vi "PF_FindExtrema.vi"(7 "Min Cut-off":sgl=0.25, 8 "Max Cut-on":sgl=0.75, 10 "Intensity Array":sgl[](array[numeric])) -> (1 "Extrema Array":T1(array[cluster]))   [LabVIEW 2019]
panel:
  in  "Extrema Cluster":T2={"type"=enum."maximum", "x"=0, "y"=0.0} {"y" format="%.2f"}
  # "Phase Fitter: Find Extrema"
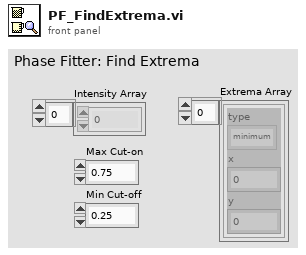
[diagram p1: front panel]
types:
  T1 = cluster{"type":enum16{"minimum", "maximum"}, "x":i32, "y":dbl}[]
  T2 = cluster{"type":enum16{"minimum", "maximum"}, "x":i32, "y":dbl}
  T3 = cluster{"Extremum":enum16{"minimum", "maximum"}, i32, sgl}
  T4 = cluster{"Extremum":enum16{"minimum", "maximum"}, "x":i32, "y":dbl}[]
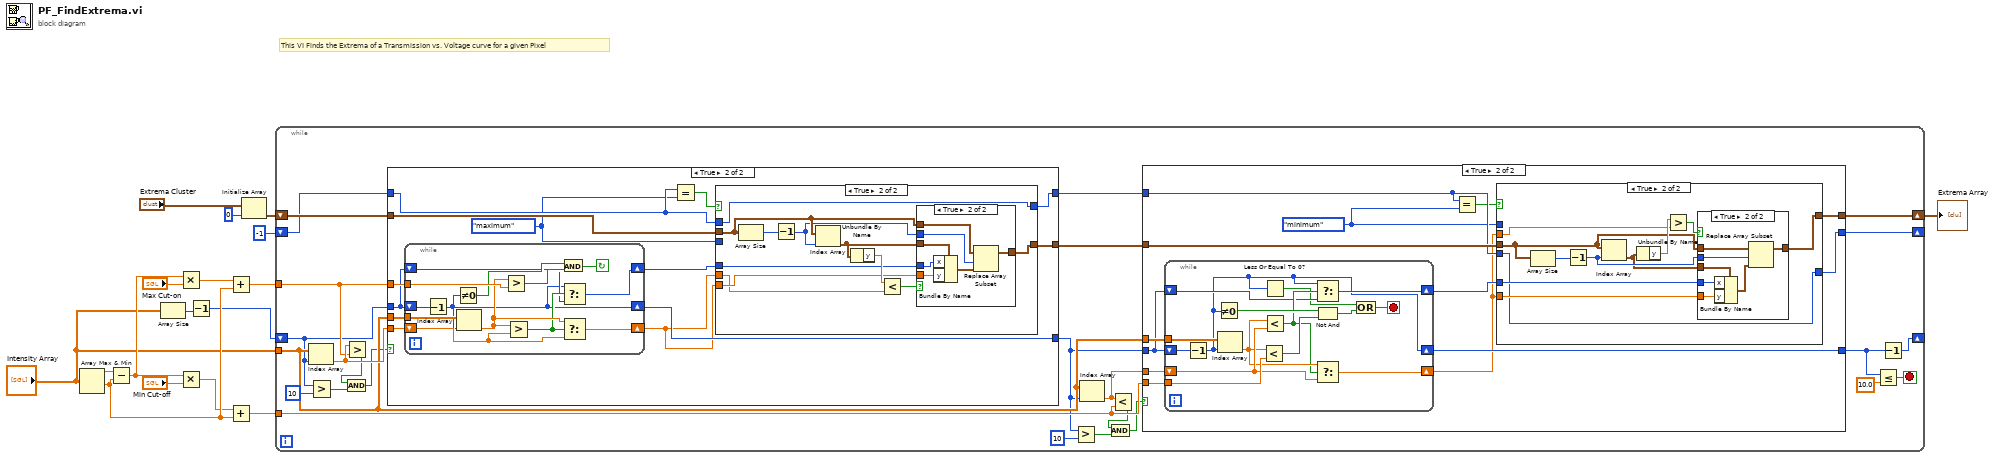
[diagram p0: block diagram]
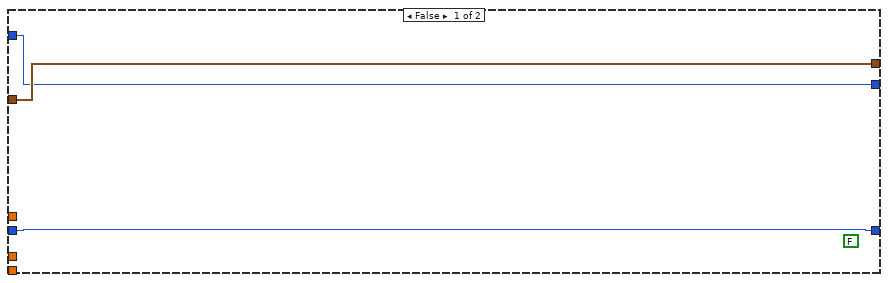
[diagram p2: hidden frame]
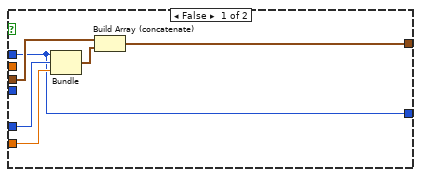
[diagram p3: hidden frame]
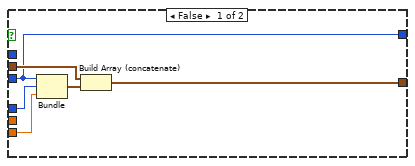
[diagram p6: hidden frame]
diagram:
  # "This VI Finds the Extrema of a Transmission vs. Voltage curve for a given Pixel"
  n1 = Array Max & Min(array="Intensity Array") -> (max value=w11:sgl, min value=w15:sgl)  [unwired: 2 out]
  n2 = Subtract(x=w11, y=w15) -> (x-y=w14:sgl)
  n3 = Array Size(array="Intensity Array") -> (size(s)=w3:i32)
  n4 = Multiply(x=w14, y="Max Cut-on") -> (x*y=w12:sgl)
  n5 = Multiply(x=w14, y="Min Cut-off") -> (x*y=w13:sgl)
  n6 = Decrement(x=w3) -> (x-1=w2:i32)
  n7 = Add(x=w12, y=w15) -> (x+y=w10:sgl)
  n8 = Add(x=w13, y=w15) -> (x+y=w9:sgl)
  n9 = Initialize Array("Extrema Cluster", 0 ("Dimension Size")) -> (w16:T1)
  n10 = while {
    shift-left: -1 -> [w38]
    shift-right: [w35] -> _
    tunnel: w9 -> [w31]
    tunnel: w10 -> [w39]
    shift-left: w16 -> [w41]
    shift-right: [w34] -> w8
    tunnel: "Intensity Array" -> [w33]
    shift-left: w2 -> [w26]
    shift-right: [w40] -> _
    stop <- w29 stop-if-true
    n11 = Index Array(array=w33, index=w26) -> (element=w42:sgl)
    n12 = Greater?(x=w26, y=10) -> (0:w27:bool)
    n13 = Greater?(x=w42, y=w39) -> (0:w24:bool)
    n14 = And(x=w24, y=w27) -> (x .and. y?=w23:bool)
    n15 = case shown="True" w23 {
      tunnel: w33 -> [_ w114]
      tunnel: w26 -> [w101 w111]
      tunnel: [w101 w112] -> w21
      tunnel: w39 -> [_ w113]
      tunnel: w42 -> [_ w110]
      tunnel: w41 -> [w100 w108]
      tunnel: [w100 w107] -> w36
      tunnel: w38 -> [w99 w105]
      tunnel: [w99 w106] -> w37
      frame False {
      }
      frame True {
        w104 = enum16{"minimum", "maximum"}."maximum" ("Extremum")
        n16 = while {
          shift-left: w111 -> [w116]
          shift-right: [w117] -> w109
          shift-left: w110 -> [w124]
          shift-right: [w123] -> w102
          tunnel: w113 -> [w125]
          shift-left: w111 -> [w127]
          shift-right: [w115] -> w112
          tunnel: w114 -> [w126]
          stop <- w120 continue-if-true
          n17 = Decrement(x=w127) -> (x-1=w115:i32)
          n18 = Not Equal To 0?(x=w115) -> (x != 0?=w122:bool)
          n19 = Index Array(array=w126, index=w115) -> (element=w119:sgl)
          n20 = Greater?(x=w119, y=w125) -> (0:w121:bool)
          n21 = Greater?(x=w119, y=w124) -> (0:w118:bool)
          n22 = And(x=w122, y=w121) -> (x .and. y?=w120:bool)
          n23 = Select(t=w115, s=w118, f=w116) -> (s? t:f=w117:i32)
          n24 = Select(t=w119, s=w118, f=w124) -> (s? t:f=w123:sgl)
        }
        n25 = Equal?(x=w105, y=w104) -> (x = y?=w103:bool)
        n26 = case shown="True" w103 {
          tunnel: w109 -> [w131 w136]
          tunnel: w108 -> [w133 w141]
          tunnel: [w132 w139] -> w107
          tunnel: w102 -> [w130 w142]
          tunnel: w105 -> [_ w134]
          tunnel: [w128 w134] -> w106
          tunnel: w104 -> [w128 _]
          tunnel: w102 -> [_ w138]
          frame False {
            n27 = Bundle("Extremum"=w128, w131, w130) -> (w129:T3)  [unwired: 1 out]
            n28 = Build Array (concatenate)(w133, w129) -> (w132:T4)
          }
          frame True {
            n29 = Array Size(array=w141) -> (size(s)=w144:i32)
            n30 = Decrement(x=w144) -> (x-1=w137:i32)
            n31 = Index Array(array=w141, index=w137) -> (element=w135:T2)
            n32 = Unbundle By Name(w135) -> ("y"=w143:dbl)
            n33 = Less?(x=w143, y=w138) -> (x < y?=w140:bool)
            n34 = case shown="True" w140 {
              tunnel: w141 -> [w145 w152]
              tunnel: [w145 w151] -> w139
              tunnel: w137 -> [_ w150]
              tunnel: w136 -> [_ w147]
              tunnel: w142 -> [_ w146]
              tunnel: w135 -> [_ w149]
              frame False {
              }
              frame True {
                n35 = Bundle By Name(cluster=w149, "x"=w147, "y"=w146) -> (w148:T2)
                n36 = Replace Array Subset(array=w152, new element=w148, index=w150) -> (w151:T1)
              }
            }
          }
        }
      }
    }
    n37 = Greater?(x=w21, y=10) -> (0:w22:bool)
    n38 = Index Array(array=w33, index=w21) -> (element=w32:sgl)
    n39 = Less?(x=w32, y=w31) -> (x < y?=w19:bool)
    n40 = And(x=w19, y=w22) -> (x .and. y?=w18:bool)
    n41 = case shown="True" w18 {
      tunnel: w33 -> [_ w58]
      tunnel: w21 -> [w45 w55]
      tunnel: [w45 w56] -> w28
      tunnel: w31 -> [_ w57]
      tunnel: w32 -> [_ w54]
      tunnel: w36 -> [w44 w52]
      tunnel: [w44 w51] -> w34
      tunnel: w37 -> [w43 w49]
      tunnel: [w43 w50] -> w35
      frame False {
        (unwired) FALSE ("Time has Elapsed")
      }
      frame True {
        w48 = enum16{"minimum", "maximum"}."minimum" ("Extremum")
        n42 = while {
          shift-left: w55 -> [w63]
          shift-right: [w64] -> w53
          shift-left: w54 -> [w70]
          shift-right: [w69] -> w46
          tunnel: w57 -> [w71]
          shift-left: w55 -> [w73]
          shift-right: [w60] -> w56
          tunnel: w58 -> [w72]
          stop <- w61 stop-if-true
          n43 = Decrement(x=w73) -> (x-1=w60:i32)
          n44 = Not Equal To 0?(x=w60) -> (x != 0?=w68:bool)
          n45 = Index Array(array=w72, index=w60) -> (element=w66:sgl)
          n46 = Less?(x=w66, y=w71) -> (x < y?=w67:bool)
          n47 = Less Or Equal To 0?(x=w60) -> (x <= 0?=w59:bool)
          n48 = Less?(x=w66, y=w70) -> (x < y?=w65:bool)
          n49 = Select(t=w60, s=w65, f=w63) -> (s? t:f=w64:i32)
          n50 = Not And(1:w67, 2:w68) -> (0:w62:bool)
          n51 = Select(t=w66, s=w65, f=w70) -> (s? t:f=w69:sgl)
          n52 = Compound Arithmetic op=OR(w59, w62) -> (w61:bool)
        }
        n53 = Equal?(x=w49, y=w48) -> (x = y?=w47:bool)
        n54 = case shown="True" w47 {
          tunnel: w53 -> [w77 w82]
          tunnel: w52 -> [w79 w87]
          tunnel: [w78 w85] -> w51
          tunnel: w46 -> [w76 w88]
          tunnel: w49 -> [_ w80]
          tunnel: [w74 w80] -> w50
          tunnel: w48 -> [w74 _]
          tunnel: w46 -> [_ w84]
          frame False {
            n55 = Bundle("Extremum"=w74, w77, w76) -> (w75:T3)  [unwired: 1 out]
            n56 = Build Array (concatenate)(w79, w75) -> (w78:T4)
          }
          frame True {
            n57 = Array Size(array=w87) -> (size(s)=w90:i32)
            n58 = Decrement(x=w90) -> (x-1=w83:i32)
            n59 = Index Array(array=w87, index=w83) -> (element=w81:T2)
            n60 = Unbundle By Name(w81) -> ("y"=w89:dbl)
            n61 = Greater?(x=w89, y=w84) -> (0:w86:bool)
            n62 = case shown="True" w86 {
              tunnel: w87 -> [w91 w98]
              tunnel: [w91 w97] -> w85
              tunnel: w83 -> [_ w96]
              tunnel: w82 -> [_ w93]
              tunnel: w88 -> [_ w92]
              tunnel: w81 -> [_ w95]
              frame False {
              }
              frame True {
                n63 = Bundle By Name(cluster=w95, "x"=w93, "y"=w92) -> (w94:T2)
                n64 = Replace Array Subset(array=w98, new element=w94, index=w96) -> (w97:T1)
              }
            }
          }
        }
      }
    }
    n65 = Less Or Equal?(x=w28, y=10.0) -> (x <= y?=w29:bool)
    n66 = Decrement(x=w28) -> (x-1=w40:i32)
  }
  "Extrema Array" <- w8
